vi "BRig_dataTrial_L_Cue2_trig_n_l2.vi"() -> (2 "output_L_Cue2_trig_n_l2":i32)   [LabVIEW 2014]
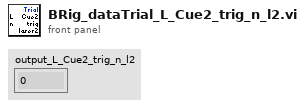
[diagram p1: front panel]
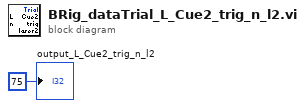
[diagram p0: block diagram]
diagram:
  "output_L_Cue2_trig_n_l2" <- 75 ("output_iBlock")
